vi "Endpoint-Load Config.vi"(8 "Error In":errorcluster) -> (0 "Error Out":errorcluster, 3 "Endpoint Config":T1[](array[typedef]))   [LabVIEW 2020]
uses:
  Endpoint-Spec.ctl
  Endpoint-Modality.ctl
  Endpoint-Laterality.ctl
  <vilib>/Utility/sysdir.llb/System Directory Type.ctl
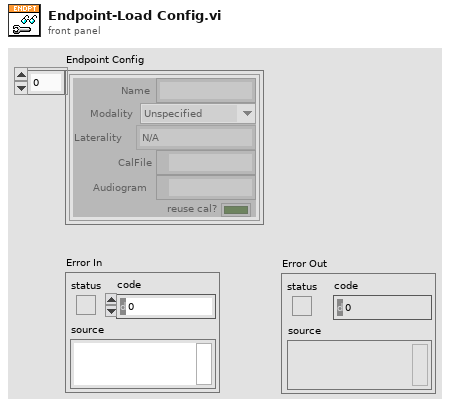
[diagram p1: front panel]
types:
  T1 = typedef "Endpoint-Spec.ctl" = cluster{"Name":string, "Modality":T2, "Laterality":T3, "CalFile":path, "Audiogram":path, "reuse cal?":bool}
  T2 = typedef "Endpoint-Modality.ctl" = enum16{"Unspecified", "Acoustic", "Electric", "Optical"}
  T3 = typedef "Endpoint-Laterality.ctl" = enum16{"N/A", "Right", "Left"}
  T4 = typedef "System Directory Type.ctl" = i32
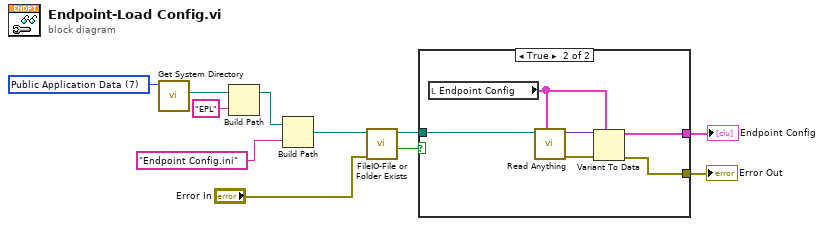
[diagram p0: block diagram]
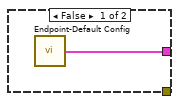
[diagram p2: hidden frame]
diagram:
  w11 = T4 7 items=["User Home"=0, "User Desktop"=1, "User Documents"=2, "User Application Data"=3, "User Preferences"=4, "User Temporary"=5, "Public Documents"=6, "Public Application Data"=7, "Public Preferences"=8, "Public Cache"=13, "System Core Libraries"=9, "System Installed Libraries"=10, "Application Files"=11, "Boot Volume Root"=12] ("system directory type")
  n1 = call <vilib>:"Get System Directory.vi"("system directory type"=w11) -> ("system directory"=w10:path)  [unwired: 10 in]
  n2 = Build Path(base path=w10, name or relative path="EPL") -> (appended path=w2:path)
  n3 = Build Path(base path=w2, name or relative path="Endpoint Config.ini") -> (appended path=w5:path)
  n4 = call "FileIO-File or Folder Exists.vi"("error in (no error)"="Error In", "path"=w5) -> ("Exists?"=w4:bool, "dup path"=w3:path)  [unwired: 6 in, 2 out]
  n5 = case shown="True" w4 {
    tunnel: [w12 w15] -> w8
    tunnel: [_ w14] -> w7
    tunnel: w3 -> [_ w13]
    frame False {
      n6 = call "Endpoint-Default Config.vi"() -> ("Default Endpoint Config"=w12:T1[])  [unwired: 1 in]
    }
    frame True {
      n7 = local read "Endpoint Config"() -> (w16:T1[])
      n8 = call "Read Anything.vi"("Type of Anything"=w16, "Path (dialog)"=w13) -> ("Error Out"=w18:errorcluster, "Anything"=w17:variant)  [unwired: 7 in, 1 out]
      n9 = Variant To Data(error in=w18, type=w16, Variant=w17) -> (data=w15:T1[], error out=w14:errorcluster)
    }
  }
  "Endpoint Config" <- w8
  "Error Out" <- w7
